vi "Set Move Right Defaults.vi"(4 "Units":string="mm", 6 "Speed":dbl=25.0, 8 "error in":errorcluster, 11 "Object":string="Base") -> (0 "error out":errorcluster)   [LabVIEW 2013]
uses:
  Arm Globals.vi
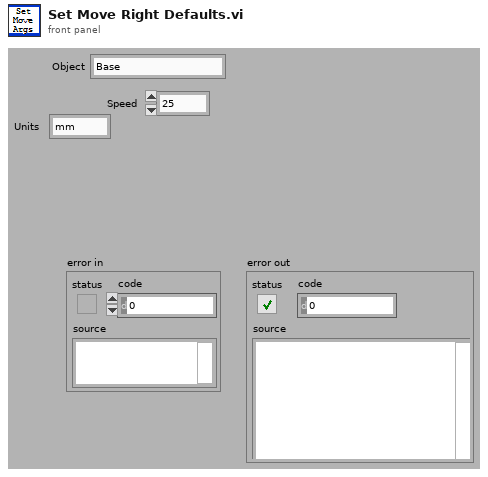
[diagram p1: front panel]
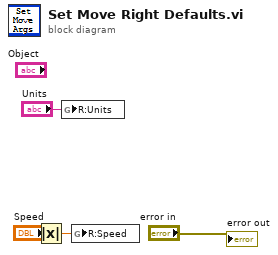
[diagram p0: block diagram]
diagram:
  n1 = Absolute Value(x="Speed") -> (abs(x)=w1:dbl)
  n2 = global write "Arm Globals.vi" "R:Units"("Units") -> ()
  n3 = global write "Arm Globals.vi" "R:Speed"(w1) -> ()
  "error out" <- "error in"
